vi "StatusUpdate.vi"   [LabVIEW 2019]
uses:
  StringUtilities/StringUtilities.lvlib
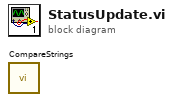
[diagram p0: block diagram]
diagram:
  n1 = call "CompareStrings.vi"() -> ()  [unwired: 12 in]
